vi "Actor Core.vi"(8 "error in":errorcluster, 11 "RUS Measurement in":refnum<class "RUS Measurement.lvclass">) -> (0 "error out":errorcluster, 3 "Actor out":refnum<class "Actor.lvclass">)   [LabVIEW 2015, in "RUS Measurement.lvclass"]
doc: "(<B>Filename</B>: Actor Framework.lvlib:Actor.lvclass:Actor Core.vi)\n\nReceives messages to the actor, reacts to them, and initiates any error handling that may shut the actor down.\n\nDescendant classes may override this VI to append parallel tasks for the actor to complete while it handles messages. Overrides use the Call Parent Method node."
uses:
  RUS Measurement.lvclass
  <vilib>/ActorFramework/Actor/Actor.lvclass
  RUS Parameters.ctl
  Controls/Menu object.ctl
  RUS Measurement.lvclass/RUS Measurement.ctl
  Mag Lab Root/Mag Lab Root.lvclass/Mag Lab Root.ctl
  <vilib>/ActorFramework/Actor/Actor.lvclass/Actor.ctl
  Mag Lab Measure Base Messages/Open sub-object parameters Msg/Open nested object parameters Msg.lvclass/Open nested object parameters Msg.ctl
  <vilib>/ActorFramework/Message Enqueuer/Message Enqueuer.lvclass/Message Enqueuer.ctl
  Read RUS Instruments.vi
  Write Instrument ref.vi
  <vilib>/ActorFramework/Message Enqueuer/Init from Existing Queue.vi
  <vilib>/ActorFramework/Message Enqueuer/Enqueue.vi
  <vilib>/ActorFramework/Message Priority Queue/Priority Enqueue.vi
  <vilib>/ActorFramework/Message Enqueuer/Message Enqueuer.lvclass
  Mag Lab Measure Base Messages/Open sub-object parameters Msg/Open nested object parameters Msg.lvclass
  Mag Lab Measurement/Mag Lab Measurement.lvclass
  Mag Lab Root/Mag Lab Root.lvclass
  Mag Lab Error Handler/Mag Lab Error Handler.lvclass
panel:
  in  "RUS Instrument":T1 {"Object name" items=["Select one"]}
  in  "Parameters":T2={"Start frequency"=790000.0, "End frequency"=810000.0, "Duration"=40.0, "Averaging"=0.0084, "Find peaks"=FALSE} {"Averaging" format="%#_6p"; "Duration" format="%#_6p"; "End frequency" format="%#_6p"; "Start frequency" format="%#_6p"}
  # "Hz"
  # "s"
  # "Hz"
  # "s"
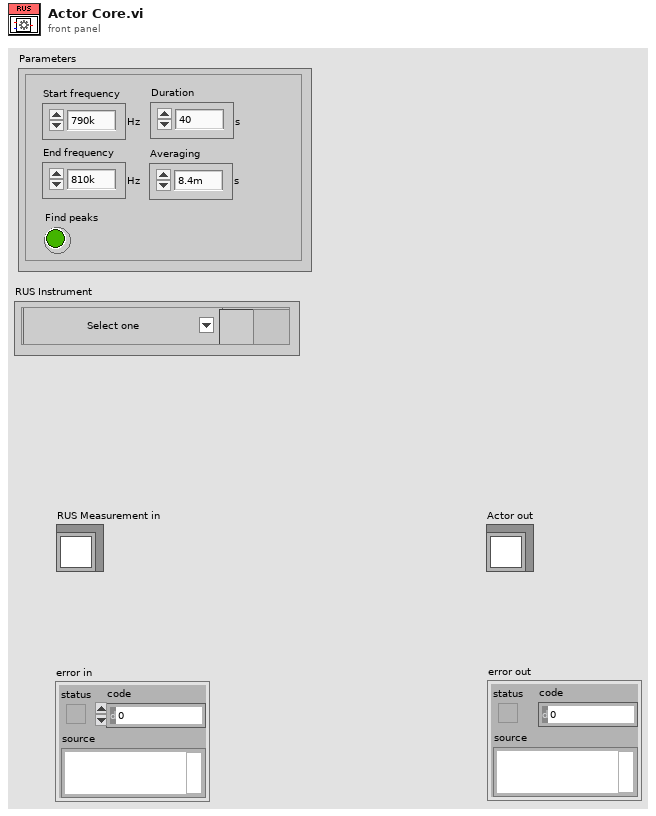
[diagram p1: front panel]
types:
  T1 = typedef "Menu object.ctl" = cluster{"Object name":u16, "Open parameters":bool, "Remove Button":bool}
  T2 = typedef "RUS Parameters.ctl" = cluster{"Start frequency":dbl, "End frequency":dbl, "Duration":dbl, "Averaging":dbl, "Find peaks":bool}
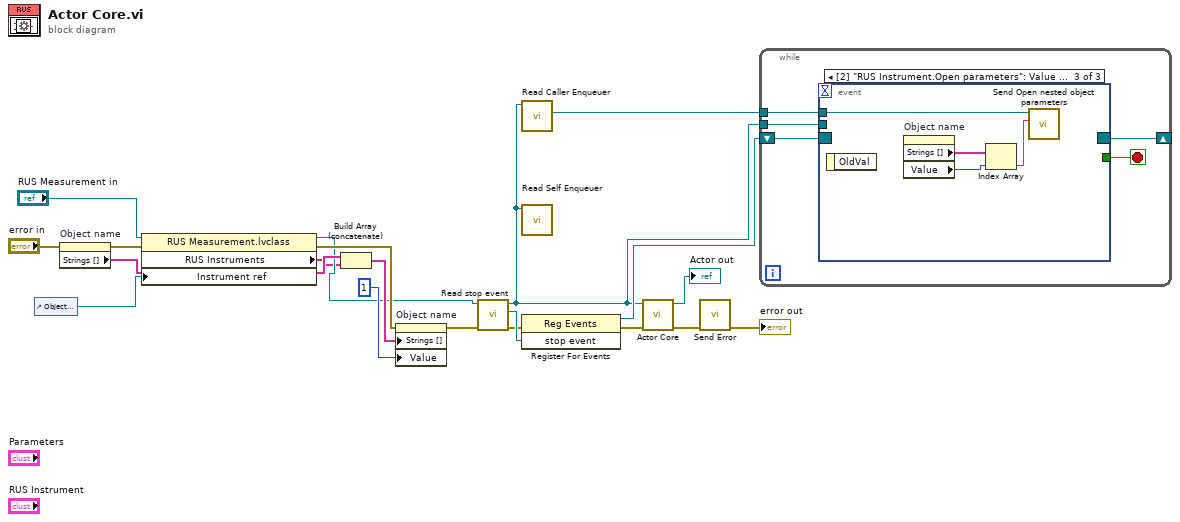
[diagram p0: block diagram]
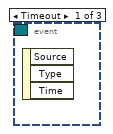
[diagram p2: hidden frame]
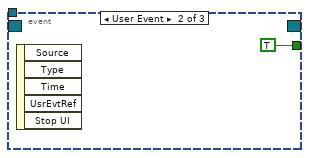
[diagram p3: hidden frame]
diagram:
  n1 = control-ref of="Object name"() -> (w1:refnum<vi>)
  n2 = property on="Object name" class="Ring (strict)"(error in="error in") -> (error out=w7:errorcluster, "Strings []"=w10:string[])  [unwired: 1 in, 1 out]
  n3 = property class="RUS Measurement.lvclass"(reference="RUS Measurement in", error in=w7, "Instrument ref"=w1) -> (reference out=w3:refnum<class "RUS Measurement.lvclass">, error out=w6:errorcluster, "RUS Instruments"=w2:string[])
  n4 = Build Array (concatenate)(w10, w2) -> (w5:string[])
  n5 = property on="Object name" class="Ring (strict)"(error in=w6, "Strings []"=w5, "Value"=u16 1) -> (error out=w8:errorcluster)  [unwired: 1 in, 1 out]
  n6 = call "Read stop event.vi"("error in (no error)"=w8, "Mag Lab Root in"=w3) -> ("error out"=w19:errorcluster, "stop event"=w20:refnum<user-event>, "Mag Lab Root out"=w12:refnum<class "RUS Measurement.lvclass">)  [unwired: 7 in]
  n7 = call <vilib>:"Read Caller Enqueuer.vi"("Actor"=w12) -> ("Caller Enqueuer"=w11:refnum<class "Message Enqueuer.lvclass">)  [unwired: 10 in]
  n8 = call <vilib>:"Read Self Enqueuer.vi"("Actor"=w12) -> ()  [unwired: 10 in, 1 out]
  n9 = register-events(error in=w19, w20) -> (reference out=w17:refnum<event-registration>, error out=w16:errorcluster)  [unwired: 1 in]
  n10 = call-parent "Actor Core.vi"("error in"=w16, "Mag Lab Measure Base in"=w12) -> ("error out"=w15:errorcluster, "Actor out"=→"Actor out":refnum<class "Actor.lvclass">)  [unwired: 8 in]
  n11 = call "Send Error.vi"("error in (no error)"=w15) -> ("error out"=→"error out":errorcluster)  [unwired: 9 in, 1 out]
  n12 = while {
    shift-right: [w24] -> _
    shift-left: w17 -> [w25]
    tunnel: w12 -> [w22]
    tunnel: w11 -> [w21]
    stop <- w23 stop-if-true
    n13 = event shown="[2] \"RUS Instrument.Open parameters\": Value Change" {
      selector: w25 -> [_ _ _]
      dyn-events: [_ _ _] -> w24
      timeout: _ -> [_ _ _]
      tunnel: [_ TRUE _] -> w23
      tunnel: w22 -> [_ _ _]
      tunnel: w21 -> [_ _ w27]
      event Timeout {
        n14 = event-data() -> ()  [unwired: 1 in, 3 out]
      }
      event User Event {
        n15 = event-data() -> ()  [unwired: 1 in, 5 out]
      }
      event Value Change {
        n16 = event-data() -> ()  [unwired: 1 in, 1 out]
        n17 = property on="Object name" class="Ring (strict)"() -> ("Strings []"=w30:string[], "Value"=w29:u16)  [unwired: 2 in, 2 out]
        n18 = Index Array(array=w30, index=w29) -> (element=w28:string)
        n19 = call "Send Open nested object parameters.vi"("Object name"=w28, "Message Enqueuer"=w27) -> ()  [unwired: 8 in, 2 out]
      }
    }
  }
